vi "Construct ConsoleView.vi"(8 "error in (no error)":errorcluster, 10 "Persist after shutdown?":bool, 11 "StringFormat":refnum<class "IStringFormat.lvclass">) -> (0 "error out":errorcluster, 3 "ConsoleView out":refnum<class "ConsoleView.lvclass">)   [LabVIEW 2017, in "ConsoleView.lvlib" / "ConsoleView.lvclass"]
uses:
  <vilib>/gpm_packages/@cs/event-logger/Source/ConsoleView/View/ConsoleView.lvclass
  <vilib>/gpm_packages/@cs/event-logger/Source/IStringFormat/IStringFormat.lvclass
  <vilib>/gpm_packages/@cs/event-logger/Source/ConsoleView/View/ConsoleView.lvclass/ConsoleView.ctl
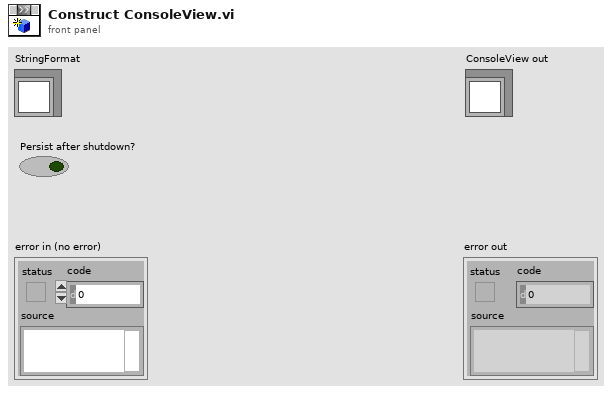
[diagram p1: front panel]
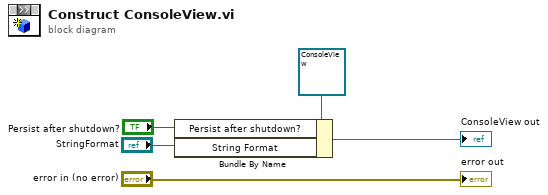
[diagram p0: block diagram]
diagram:
  n1 = Bundle By Name(cluster=refnum<class "ConsoleView.lvclass"> refnum ("ConsoleView Sink in"), "Persist after shutdown?"="Persist after shutdown?", "String Format"="StringFormat") -> (→"ConsoleView out":refnum<class "ConsoleView.lvclass">)
  "error out" <- "error in (no error)"
